vi "Fire Control Loop.vi"(4 "Prime BB DevRef":T5, 6 "OnDeck BB DevRef":T5, 7 "Fire Log Enable":bool=TRUE, 8 "FireDevRef":T7={"DevStatus"={"status"=FALSE, "code"=0, "source"=""}, "Solenoid Module"=enum."Solenoid Module 1", "Forward Solenoid Channel"=enum."Invalid", "Reverse Solenoid Channel"=enum."Invalid"}, 9 "Time Ref":dbl, 10 "ConveyorDevRef":T1, 11 "rt fifo":refnum<k33>, 12 "Fire State In":T10, 13 "LogArray":i32[](array[numeric]), 14 "iteration":i32, 15 "IndexerDevRef":T7={"DevStatus"={"status"=FALSE, "code"=0, "source"=""}, "Solenoid Module"=enum."Solenoid Module 1", "Forward Solenoid Channel"=enum."Invalid", "Reverse Solenoid Channel"=enum."Invalid"}) -> (0 "Fire":bool, 1 "Fire State Out":T10, 3 "# elements":u32)   [LabVIEW 2012]
uses:
  <vilib>/Rock Robotics/WPI/Solenoid/WPI_SolenoidValue.ctl
  fire_step_state.ctl
  <vilib>/Rock Robotics/WPI/Solenoid/WPI_SolenoidDevRef.ctl
  <vilib>/Rock Robotics/SystemInterfaces/Typedef/FPGA_TypedefSolenoidModule.ctl
  <vilib>/Rock Robotics/WPI/Solenoid/WPI_SolenoidChannel.ctl
  <vilib>/Rock Robotics/WPI/DigitalInput/WPI_DigitalInputDevRef.ctl
  <vilib>/Rock Robotics/SystemInterfaces/DIO/FPGA_DIOChannel.ctl
  <vilib>/Rock Robotics/SystemInterfaces/Typedef/FPGA_TypedefDigitalModule.ctl
  <vilib>/Rock Robotics/WPI/Relay/WPI_RelayDevRef.ctl
  <vilib>/Rock Robotics/SystemInterfaces/DIO/FPGA_DIORelayChannel.ctl
  <vilib>/Rock Robotics/WPI/Relay/WPI_RelayDirection.ctl
  <vilib>/Rock Robotics/WPI/DriverStation/WPI_DriverStationRobotMode2.ctl
  <vilib>/Rock Robotics/WPI/Relay/WPI_RelayValue.ctl
  <vilib>/Rock Robotics/WPI/Solenoid/WPI_SolenoidSetEnum.vi
panel:
  in  "test stable":bool
  in  "Pusher On":bool=TRUE
  in  "Sample Rate (sec) 5":dbl=1.0
  in  "Width (sec)":dbl=0.1
  out "Wish":dbl
  in  "Test Ind":T11
  out "Cmd":T11
  out "Air Lock":bool
  out "Prime":bool
  out "OnDeck":bool
  in  "Prime arrive delay":dbl=0.1
  in  "Prime depart delay":dbl=0.1
  in  "AL arrive delay":dbl
  in  "AL depart delay":dbl
  in  "OD Delay":dbl=0.2
  in  "OD Width":dbl=0.15
  out "Prime":cluster{i16, i16}(graph)
  out "On Deck":cluster{i16, i16}(graph)
  # "Prime Rising edge: Delay Indexer Back-to-Front action to allow\ntime for Disc to drop before allowing next Disc into 'AirLock'.\n(Anytime Indexer is 'Back', it means a Disc is on it's way to drop.)\nIf this delay not required, set to minimum necessary to reliably\ndebounce Rising Edge transition."
  # "Fire Solenoid"
  # "Solenoid Test"
  # "Prime Falling edge: Delay Indexer Front-to-Back action to allow\ntime for Prime Disc to depart and Kicker to reset before allowing\nnext Disc out of 'AirLock' to drop into Prime.\nThis time is in parallel with Disc motion from AirLock and any\nOnDeck Rising Edge delay/debounce.\nIf this delay not required, set to minimum necessary to reliably\ndebounce Falling Edge transition."
  # "OnDeck Rising edge: Delay Indexer Front-to-Back action to allow\ntime for disc to get inside AirLock without back door collision.\nIf this delay not required, set to minimum necessary to reliably\ndebounce Rising Edge transition."
  # "Use to delay OD\nResponse"
  # "Use to normalize OD\npulse"
  # "OnDeck Falling edge: Falling edge has no control impact given \ncurrent state machine design - no physical implication.\nSet to minimum necessary to reliably debounce Falling Edge\ntransition, as best practice."
  # "TDMS"
  # "Off will Disable\nOn will :\n   if Robot Mode is Disabled\n      log at Sample Rate\n    else\n      log Continuously"
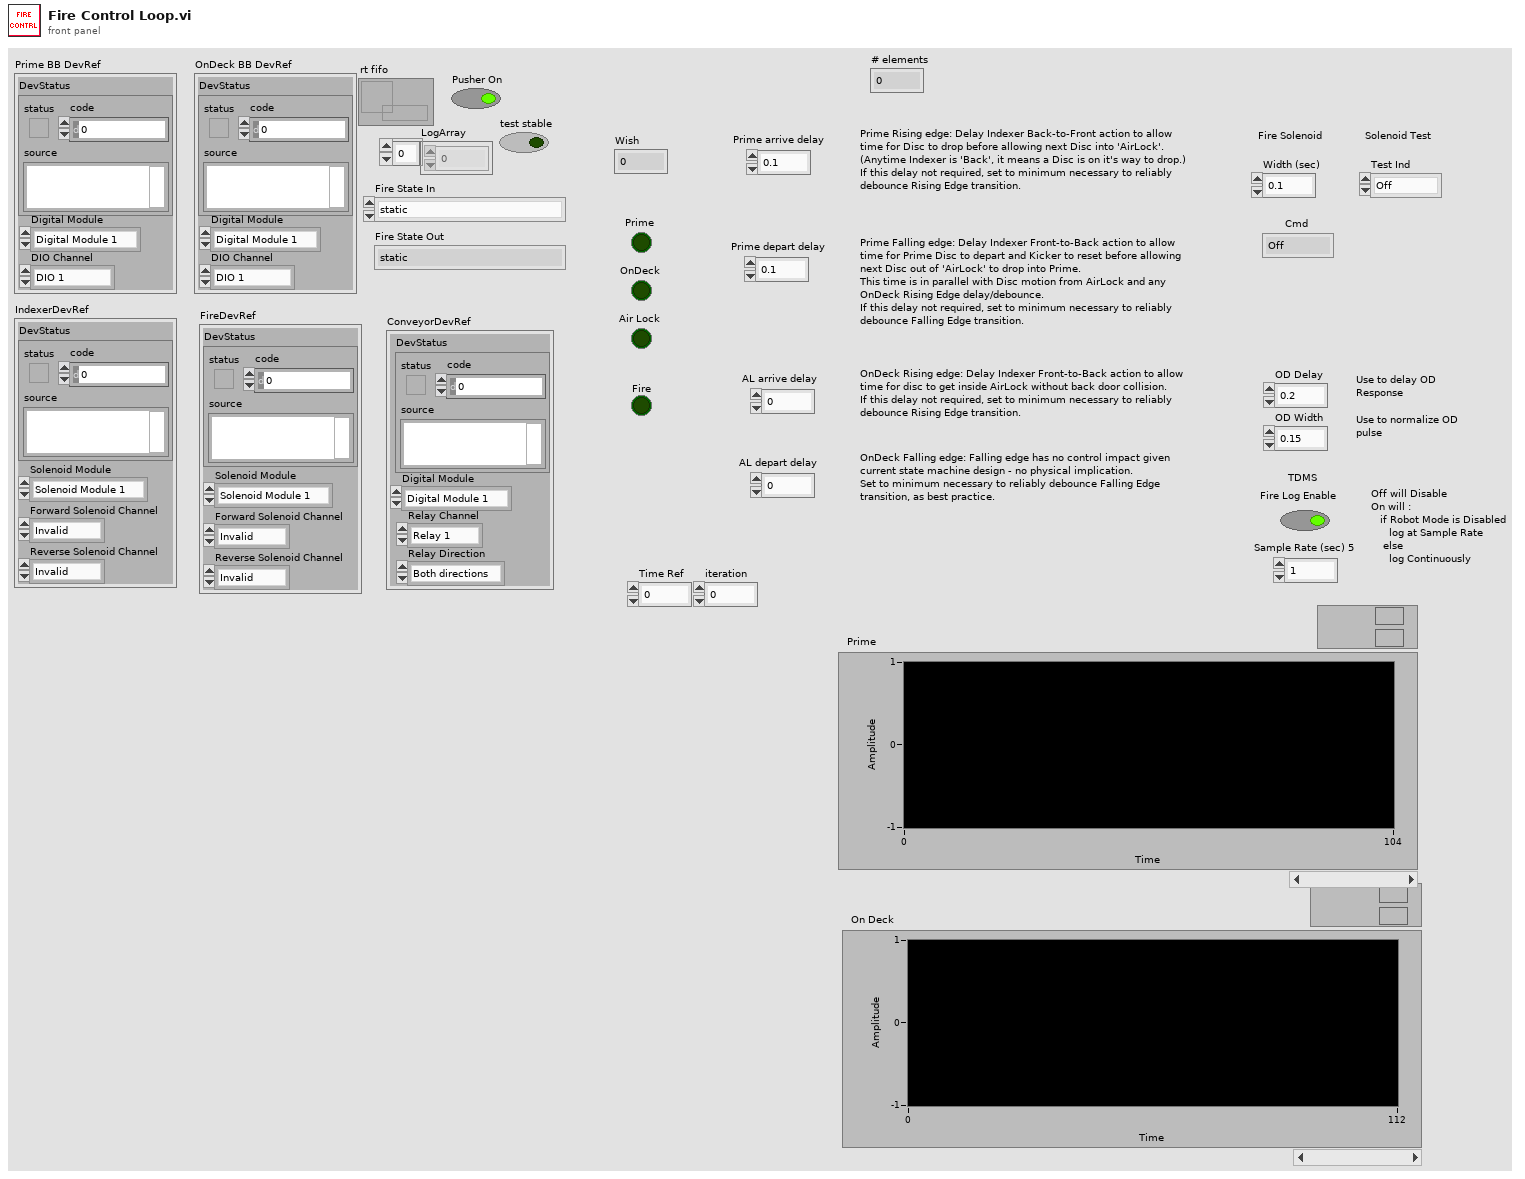
[diagram p1: front panel]
types:
  T1 = typedef "WPI_RelayDevRef.ctl" = cluster{"DevStatus":errorcluster, "Relay Channel":T2, "Digital Module":T3, "Relay Direction":T4}
  T2 = typedef "FPGA_DIORelayChannel.ctl" = enum8{"Relay 1", "Relay 2", "Relay 3", "Relay 4", "Relay 5", "Relay 6", "Relay 7", "Relay 8", "Invalid"}
  T3 = typedef "FPGA_TypedefDigitalModule.ctl" = enum16{"Digital Module 1", "Digital Module 2"}
  T4 = typedef "WPI_RelayDirection.ctl" = enum16{"Both directions", "Forward only", "Reverse only"}
  T5 = typedef "WPI_DigitalInputDevRef.ctl" = cluster{"DevStatus":errorcluster, "DIO Channel":T6, "Digital Module":T3}
  T6 = typedef "FPGA_DIOChannel.ctl" = enum8{"DIO 1", "DIO 2", "DIO 3", "DIO 4", "DIO 5", "DIO 6", "DIO 7", "DIO 8", "DIO 9", "DIO 10", "DIO 11", "DIO 12", "DIO 13", "DIO 14", "Invalid"}
  T7 = typedef "WPI_SolenoidDevRef.ctl" = cluster{"DevStatus":errorcluster, "Solenoid Module":T8, "Forward Solenoid Channel":T9, "Reverse Solenoid Channel":T9}
  T8 = typedef "FPGA_TypedefSolenoidModule.ctl" = enum16{"Solenoid Module 1", "Solenoid Module 2"}
  T9 = typedef "WPI_SolenoidChannel.ctl" = enum8{"Solenoid 1", "Solenoid 2", "Solenoid 3", "Solenoid 4", "Solenoid 5", "Solenoid 6", "Solenoid 7", "Solenoid 8", "Invalid"}
  T10 = typedef "fire_step_state.ctl" = enum16{"static", "manual", "saftey_down", "saftey_up", "check_saftey", "fire"}
  T11 = typedef "WPI_SolenoidValue.ctl" = enum16{"Off", "On", "Forward", "Reverse"}
  T12 = typedef "WPI_DriverStationRobotMode2.ctl" = enum16{"Autonomous Disabled", "Autonomous Enabled", "Teleop Disabled", "Teleop Enabled", "Timeout", "Finish", "Test Disabled", "Test Enabled"}
  T13 = typedef "WPI_RelayValue.ctl" = enum16{"Off", "On", "Forward", "Reverse"}
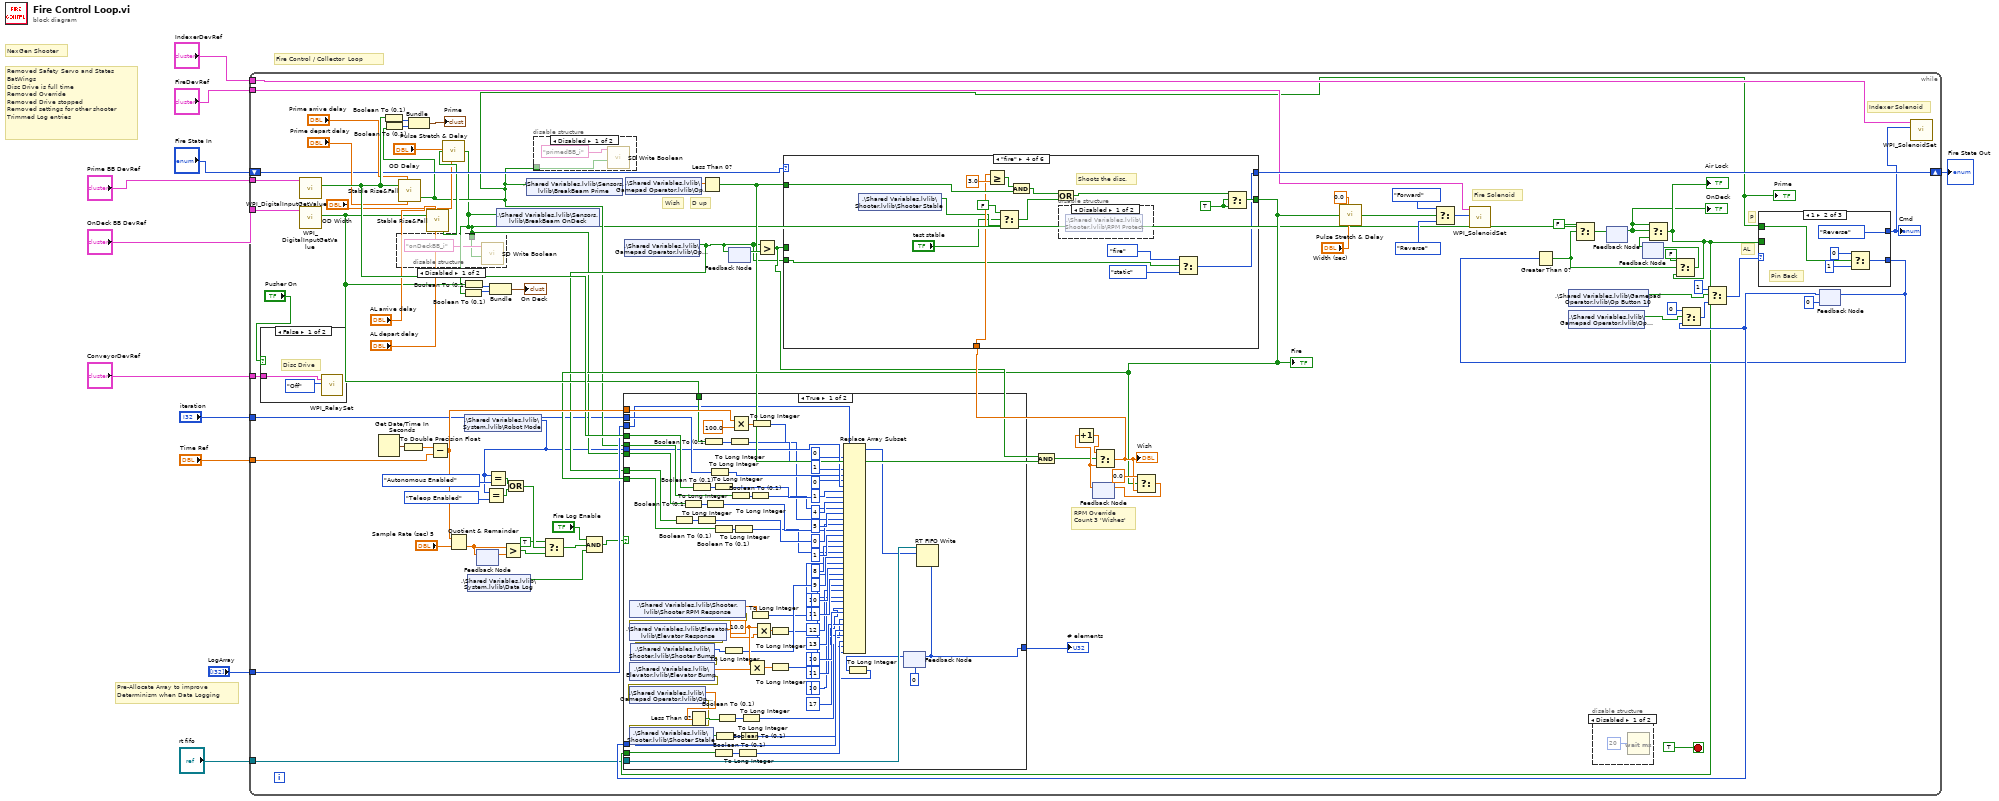
[diagram p0: block diagram]
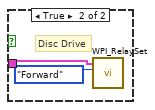
[diagram p2: hidden frame]
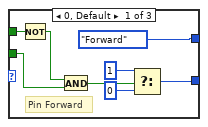
[diagram p6: hidden frame]
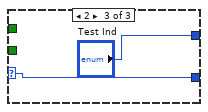
[diagram p7: hidden frame]
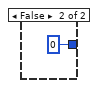
[diagram p8: hidden frame]
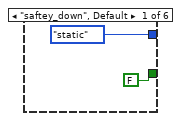
[diagram p9: hidden frame]
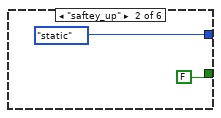
[diagram p10: hidden frame]
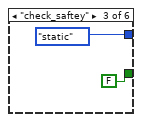
[diagram p11: hidden frame]
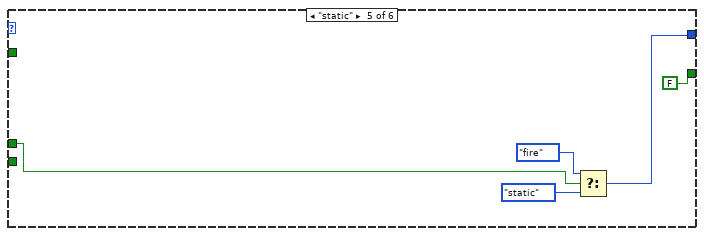
[diagram p13: hidden frame]
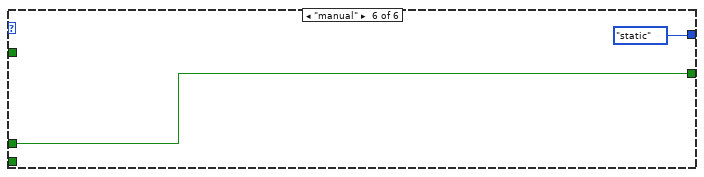
[diagram p14: hidden frame]
diagram:
  # "Pre-Allocate Array to improve \nDeterminism when Data Logging"
  # "Removed Safety Servo and States\nBatWings\nDisc Drive is full time\nRemoved Override\nRemoved Drive stopped\nRemoved settings for other shooter\nTrimmed Log entries"
  # "NexGen Shooter"
  # "Fire Control / Collector  Loop"
  n1 = while {
    tunnel: "FireDevRef" -> [w73]
    tunnel: "OnDeck BB DevRef" -> [w96]
    tunnel: "Prime BB DevRef" -> [w95]
    shift-right: [w92] -> w11
    shift-left: "Fire State In" -> [w34]
    tunnel: "Time Ref" -> [w52]
    tunnel: "IndexerDevRef" -> [w59]
    tunnel: "ConveyorDevRef" -> [w26]
    tunnel: "LogArray" -> [w25]
    tunnel: "rt fifo" -> [w16]
    tunnel: "iteration" -> [w12]
    stop <- TRUE stop-if-true
    # "Wish"
    # "D up"
    # "Indexer Solenoid"
    # "AL"
    # "P"
    # "RPM Override\nCount 3 'Wishes'"
    # "Fire Solenoid"
    n2 = case shown="False" "Pusher On" {
      tunnel: w26 -> [w97 w99]
      frame False {
        # "Disc Drive"
        n3 = call <vilib>:"WPI_RelaySet.vi"("RelayValue"=WPI_RelayValue."Off", "RelayDevRef"=w97) -> ()  [unwired: 8 in, 2 out]
      }
      frame True {
        # "Disc Drive"
        n4 = call <vilib>:"WPI_RelaySet.vi"("RelayValue"=WPI_RelayValue."Forward", "RelayDevRef"=w99) -> ()  [unwired: 8 in, 2 out]
      }
    }
    n5 = call <vilib>:"WPI_DigitalInputGetValue.vi"("DigitalInputDevRef"=w95) -> ("Value"=w71:bool)  [unwired: 8 in, 2 out]
    n6 = call <vilib>:"WPI_DigitalInputGetValue.vi"("DigitalInputDevRef"=w96) -> ("Value"=w54:bool)  [unwired: 8 in, 2 out]
    n7 = Get Date/Time In Seconds() -> (seconds since 1Jan1904=w88:timestamp)
    n8 = Boolean To (0,1)(Boolean=w71) -> (0, 1=w68:i16)
    n9 = call "Stable Rise&Fall.vi"("Signal Input"=w71, "Rise Delay(sec)"="Prime arrive delay", "Fall Delay(sec)"="Prime depart delay") -> ("Stable"=w20:bool)  [unwired: 4 in]
    "Prime" <- w20
    n10 = Boolean To (0,1)(Boolean=w20) -> (0, 1=w67:i16)
    n11 = To Double Precision Float(number=w88) -> (double precision float=w87:dbl)
    n12 = Bundle(w68, w67) -> (→"Prime":cluster{i16, i16})  [unwired: 1 in]
    n13 = call "Stable Rise&Fall.vi"("Signal Input"=w54, "Rise Delay(sec)"="AL arrive delay", "Fall Delay(sec)"="AL depart delay") -> ("Stable"=w32:bool)  [unwired: 4 in]
    n14 = Subtract(x=w87, y=w52) -> (x-y=w72:dbl)
    n15 = call "Pulse Stretch & Delay.vi"("Delay (sec)"="OD Delay", "In"=w32, "Width (sec)"="OD Width") -> ("Out"=w19:bool)  [unwired: 2 in]
    n16 = disable-structure shown="Disabled" {
      disable-tunnel: w19 -> [w101 _]
      frame Disabled {
        n17 = call <vilib>:"SD Write Boolean.vi"("Boolean"=w101, "Name"="onDeckBB_i") -> ()  [unwired: 8 in, 2 out]
      }
      frame Enabled {
      }
    }
    n18 = Quotient & Remainder(x=w72, y="Sample Rate (sec) 5") -> (floor(x/y)=w91:dbl)  [unwired: 1 out]
    n19 = Boolean To (0,1)(Boolean=w19) -> (0, 1=w56:i16)
    n20 = Boolean To (0,1)(Boolean=w54) -> (0, 1=w55:i16)
    n21 = shared-variable ".\\Shared Variables.lvlib\\System.lvlib\\Robot Mode"() -> (w18:i32)  [unwired: 1 in, 1 out]
    n22 = shared-variable ".\\Shared Variables.lvlib\\System.lvlib\\Data Log"() -> (w15:bool)  [unwired: 1 in, 1 out]
    n23 = feedback #1() -> (w90:dbl)  [unwired: 1 in]
    n24 = feedback-in #1(w91) -> ()
    n25 = Equal?(x=w18, y=WPI_DriverStationRobotMode2."Teleop Enabled") -> (x = y?=w81:bool)
    n26 = Equal?(x=w18, y=WPI_DriverStationRobotMode2."Autonomous Enabled") -> (x = y?=w82:bool)
    n27 = Bundle(w55, w56) -> (→"On Deck":cluster{i16, i16})  [unwired: 1 in]
    n28 = shared-variable ".\\Shared Variables.lvlib\\Sensors.lvlib\\BreakBeam OnDeck"(w19) -> ()  [unwired: 1 in, 1 out]
    n29 = Greater?(x=w91, y=w90) -> (0:w79:bool)
    n30 = Or(x=w82, y=w81) -> (x .or. y?=w80:bool)
    n31 = shared-variable ".\\Shared Variables.lvlib\\Sensors.lvlib\\BreakBeam Prime"(w20) -> ()  [unwired: 1 in, 1 out]
    n32 = disable-structure shown="Disabled" {
      disable-tunnel: w20 -> [w103 _]
      frame Disabled {
        n33 = call <vilib>:"SD Write Boolean.vi"("Boolean"=w103, "Name"="primedBB_i") -> ()  [unwired: 8 in, 2 out]
      }
      frame Enabled {
      }
    }
    n34 = Select(t=TRUE ("f"), s=w80, f=w79) -> (s? t:f=w86:bool)
    n35 = Compound Arithmetic op=AND("Fire Log Enable", w86, w15) -> (w13:bool)
    n36 = shared-variable ".\\Shared Variables.lvlib\\Gamepad Operator.lvlib\\Op Button 6"() -> (w24:bool)  [unwired: 1 in, 1 out]
    n37 = shared-variable ".\\Shared Variables.lvlib\\Gamepad Operator.lvlib\\Op Dpad (y)"() -> (w21:dbl)  [unwired: 1 in, 1 out]
    n38 = Less Than 0?(x=w21) -> (x < 0?=w33:bool)
    n39 = feedback #2() -> (w93:bool)  [unwired: 1 in]
    n40 = feedback-in #2(w24) -> ()
    n41 = Greater?(x=w24, y=w93) -> (0:w60:bool)
    n42 = And(x=w60, y=w33) -> (x .and. y?=w62:bool)
    n43 = feedback #3() -> (w66:dbl)  [unwired: 1 in]
    n44 = Increment(x=w66) -> (x+1=w65:dbl)
    n45 = Select(t=w65, s=w62, f=w66) -> (s? t:f=w61:dbl)
    "Wish" <- w61
    n46 = case shown="\"fire\"" w34 {
      tunnel: [fire_step_state."static" ("Fire State") fire_step_state."static" ("Fire State") fire_step_state."static" ("Fire State") w211 w223 fire_step_state."static" ("Fire State")] -> w92
      tunnel: w60 -> [_ _ _ _ w224 w226]
      tunnel: [FALSE FALSE FALSE w220 FALSE w226] -> w50
      tunnel: w33 -> [_ _ _ w216 _ _]
      tunnel: w61 -> [_ _ _ w214 _ _]
      tunnel: w24 -> [_ _ _ w210 _ _]
      frame "saftey_down", Default {
      }
      frame "saftey_up" {
      }
      frame "check_saftey" {
      }
      frame "fire" {
        w209 = TRUE
        # "Shoots the disc."
        n47 = shared-variable ".\\Shared Variables.lvlib\\Shooter.lvlib\\Shooter Stable"() -> (w208:bool)  [unwired: 1 in, 1 out]
        n48 = Greater Or Equal?(x=w214, y=3.0) -> (x >= y?=w218:bool)
        n49 = Select(t=FALSE, s="test stable", f=w208) -> (s? t:f=w206:bool)
        n50 = And(x=w218, y=w216) -> (x .and. y?=w219:bool)
        n51 = Or(x=w219, y=w206) -> (x .or. y?=w215:bool)
        n52 = disable-structure shown="Disabled" {
          frame Disabled {
            n53 = shared-variable ".\\Shared Variables.lvlib\\Shooter.lvlib\\RPM Protect"() -> ()  [unwired: 1 in, 2 out]
          }
          frame Enabled {
          }
        }
        n54 = Select(t=fire_step_state."fire" ("Fire State"), s=w210, f=fire_step_state."static" ("Fire State")) -> (s? t:f=w211:T10)
        n55 = Select(t=w215, s=w209, f=w209) -> (s? t:f=w220:bool)
      }
      frame "static" {
        n56 = Select(t=fire_step_state."fire" ("Fire State"), s=w224, f=fire_step_state."static" ("Fire State")) -> (s? t:f=w223:T10)
      }
      frame "manual" {
      }
    }
    "Fire" <- w50
    n57 = Select(t=0.0, s=w50, f=w61) -> (s? t:f=w64:dbl)
    n58 = feedback-in #3(w64) -> ()
    n59 = call "Pulse Stretch & Delay.vi"("Delay (sec)"=0.0, "In"=w50, "Width (sec)"="Width (sec)") -> ("Out"=w42:bool)  [unwired: 2 in]
    n60 = Select(t=WPI_SolenoidValue."Forward" ("Value"), s=w42, f=WPI_SolenoidValue."Reverse" ("Value")) -> (s? t:f=w44:T11)
    n61 = call-poly <vilib>:"WPI_SolenoidSet.vi"("Value"=w44, "SolenoidDevRef"=w73) -> ()  [unwired: 8 in, 2 out]
    n62 = shared-variable ".\\Shared Variables.lvlib\\Gamepad Operator.lvlib\\Op Button 10"() -> (w23:bool)  [unwired: 1 in, 1 out]
    n63 = shared-variable ".\\Shared Variables.lvlib\\Gamepad Operator.lvlib\\Op Button 9"() -> (w22:bool)  [unwired: 1 in, 1 out]
    n64 = disable-structure shown="Disabled" {
      frame Disabled {
        n65 = Wait (ms)(milliseconds to wait=u32 20) -> ()  [unwired: 1 out]
      }
      frame Enabled {
      }
    }
    n66 = feedback #4() -> (w36:bool)  [unwired: 1 in]
    "OnDeck" <- w36
    n67 = feedback #5() -> (w48:bool)  [unwired: 1 in]
    n68 = Select(t=w36, s=w36, f=w48) -> (s? t:f=w40:bool)
    "Air Lock" <- w40
    n69 = feedback #6(0) -> (w46:i32)
    n70 = case shown="True" w13 {
      tunnel: w72 -> [w192 _]
      tunnel: w71 -> [w197 _]
      tunnel: w20 -> [w196 _]
      tunnel: w19 -> [w195 _]
      tunnel: w24 -> [w194 _]
      tunnel: w50 -> [w193 _]
      tunnel: w12 -> [w191 _]
      tunnel: w18 -> [w186 _]
      tunnel: w54 -> [w190 _]
      tunnel: w46 -> [w187 _]
      tunnel: w40 -> [w189 _]
      tunnel: w25 -> [w188 _]
      tunnel: w16 -> [w185 _]
      tunnel: [w124 u32 0 ("# elements")] -> w14
      frame True {
        (unwired) 0 ("index")
        (unwired) 1 ("index")
        (unwired) 0 ("index")
        (unwired) 1 ("index")
        (unwired) 0 ("index")
        (unwired) 1 ("index")
        (unwired) 0 ("index")
        (unwired) 1 ("index")
        (unwired) 0 ("index")
        w175 = 10.0 ("x")
        n71 = shared-variable ".\\Shared Variables.lvlib\\Shooter.lvlib\\Shooter RPM Response"() -> (w135:dbl, error out=w132:errorcluster)  [unwired: 1 in]
        n72 = shared-variable ".\\Shared Variables.lvlib\\Elevator.lvlib\\Elevator Response"(error in=w132) -> (w136:dbl, error out=w131:errorcluster)
        n73 = shared-variable ".\\Shared Variables.lvlib\\Shooter.lvlib\\Shooter Bump"(error in=w131) -> (w134:i64, error out=w130:errorcluster)
        n74 = shared-variable ".\\Shared Variables.lvlib\\Elevator.lvlib\\Elevator Bump"(error in=w130) -> (w137:dbl, error out=w129:errorcluster)
        n75 = shared-variable ".\\Shared Variables.lvlib\\Gamepad Operator.lvlib\\Op Dpad (y)"(error in=w129) -> (w138:dbl, error out=w128:errorcluster)
        n76 = shared-variable ".\\Shared Variables.lvlib\\Shooter.lvlib\\Shooter Stable"(error in=w128) -> (w133:bool)  [unwired: 1 out]
        n77 = Boolean To (0,1)(Boolean=w194) -> (0, 1=w178:i16)
        n78 = Boolean To (0,1)(Boolean=w195) -> (0, 1=w179:i16)
        n79 = Less Than 0?(x=w138) -> (x < 0?=w170:bool)
        n80 = Boolean To (0,1)(Boolean=w197) -> (0, 1=w181:i16)
        n81 = To Long Integer(number=w178) -> (32bit integer=w146:i32)
        n82 = Boolean To (0,1)(Boolean=w190) -> (0, 1=w172:i16)
        n83 = To Long Integer(number=w179) -> (32bit integer=w147:i32)
        n84 = To Long Integer(number=w191) -> (32bit integer=w166:i32)
        n85 = To Long Integer(number=w181) -> (32bit integer=w150:i32)
        n86 = Boolean To (0,1)(Boolean=w193) -> (0, 1=w177:i16)
        n87 = Boolean To (0,1)(Boolean=w189) -> (0, 1=w171:i16)
        n88 = Boolean To (0,1)(Boolean=w133) -> (0, 1=w173:i16)
        n89 = Boolean To (0,1)(Boolean=w170) -> (0, 1=w174:i16)
        n90 = To Long Integer(number=w134) -> (32bit integer=w142:i32)
        n91 = To Long Integer(number=w172) -> (32bit integer=w148:i32)
        n92 = Multiply(x=w192, y=100.0) -> (x*y=w182:dbl)
        n93 = Boolean To (0,1)(Boolean=w196) -> (0, 1=w180:i16)
        n94 = To Long Integer(number=w177) -> (32bit integer=w139:i32)
        n95 = To Long Integer(number=w171) -> (32bit integer=w145:i32)
        n96 = To Long Integer(number=w173) -> (32bit integer=w126:i32)
        n97 = To Long Integer(number=w174) -> (32bit integer=w144:i32)
        n98 = Multiply(x=w175, y=w137) -> (x*y=w176:dbl)
        n99 = To Long Integer(number=w180) -> (32bit integer=w149:i32)
        n100 = To Long Integer(number=w135) -> (32bit integer=w140:i32)
        n101 = To Long Integer(number=w182) -> (32bit integer=w169:i32)
        n102 = Multiply(x=w175, y=w136) -> (x*y=w184:dbl)
        n103 = To Long Integer(number=w184) -> (32bit integer=w141:i32)
        n104 = To Long Integer(number=w176) -> (32bit integer=w143:i32)
        n105 = feedback #7(u32 0 ("# elements")) -> (w123:u32)
        n106 = To Long Integer(number=w123) -> (32bit integer=w122:i32)
        n107 = Replace Array Subset(array=w188, new element #1=w169, index #1=0 ("index"), new element #2=w166, index #2=1 ("index"), new element #3=w186, index #3=2 ("index"), new element #4=w150, index #4=3 ("index"), new element #5=w149, index #5=4 ("index"), new element #6=w148, index #6=5 ("index"), new element #7=w147, index #7=6 ("index"), new element #8=w146, index #8=7 ("index"), new element #9=w139, index #9=8 ("index"), new element #10=w140, index #10=9 ("index"), new element #11=w141, index #11=10 ("index"), new element #12=w142, index #12=11 ("index"), new element #13=w143, index #13=12 ("index"), new element #14=w144, index #14=13 ("index"), new element #15=w126, index #15=14 ("index"), new element #16=w187, index #16=15 ("index"), new element #17=w145, index #17=16 ("index"), new element #18=w122, index #18=17 ("index")) -> (w127:i32[])
        n108 = RT FIFO Write(0:w185, 1:w127) -> (7:w124:u32)  [unwired: 3 in, 3 out]
        n109 = feedback-in #7(w124) -> ()
      }
      frame False {
      }
    }
    "# elements" <- w14
    n110 = Select(t=0, s=w22, f=w46) -> (s? t:f=w28:i32)
    n111 = Select(t=1, s=w23, f=w28) -> (s? t:f=w27:i32)
    n112 = case shown="1" w27 {
      selector: w27 -> [_ _ w120]
      tunnel: [w111 w116 w120] -> w41
      tunnel: [WPI_SolenoidValue."Forward" ("Value") WPI_SolenoidValue."Reverse" ("Value") "Test Ind"] -> w35
      tunnel: w20 -> [w109 w115 _]
      tunnel: w40 -> [w107 _ _]
      frame 0, Default {
        # "Pin Forward"
        n113 = Not(x=w109) -> (.not. x?=w113:bool)
        n114 = And(x=w113, y=w107) -> (x .and. y?=w108:bool)
        n115 = Select(t=1, s=w108, f=0) -> (s? t:f=w111:i32)
      }
      frame 1 {
        # "Pin Back"
        n116 = Select(t=0, s=w115, f=1) -> (s? t:f=w116:i32)
      }
      frame 2 {
      }
    }
    "Cmd" <- w35
    n117 = Greater Than 0?(x=w41) -> (x > 0?=w38:bool)
    n118 = Select(t=FALSE, s=w38, f=w19) -> (s? t:f=w37:bool)
    n119 = feedback-in #4(w37) -> ()
    n120 = Select(t=FALSE, s=w38, f=w40) -> (s? t:f=w47:bool)
    n121 = feedback-in #5(w47) -> ()
    n122 = feedback-in #6(w41) -> ()
    n123 = call-poly <vilib>:"WPI_SolenoidSet.vi"("Value"=w35, "SolenoidDevRef"=w59) -> ()  [unwired: 8 in, 2 out]
  }
  "Fire State Out" <- w11
